vi "control loop bookkeeping.vi"(4 "worker pool reference":T2, 6 "fault fifo":refnum<k33>, 8 "engine error in":errorcluster, 9 "status reporting in":T19={"late? index (bool)"=-1, "late count index (U32)"=-1, "dt (ns) index (U64)"=-1}, 10 "time data in":T1, 11 "control loop data in":T5 {"module information"."GUID"."Lo" format="%.0x"; "module information"."GUID"."Hi" format="%.0x"}) -> (0 "engine error out":errorcluster, 1 "safe state?":bool, 2 "time data out":T1, 3 "control loop data out":T5 {"module information"."GUID"."Lo" format="%.0x"; "module information"."GUID"."Hi" format="%.0x"})   [LabVIEW 2013, in "main engine.lvlib"]
doc: "This VI writes to any of the timing or error tags that have been configured based on the results of this iteration of the loop."
uses:
  main engine/main engine.lvlib
  status reporting data.ctl
  control loop data.ctl
  <vilib>/NI/Tag Bus/table/data table.ctl
  engine run schedule.ctl
  engine decimation schedule.ctl
  full module data.ctl
  <vilib>/NI/Tag Bus Module Framework/runtime/TBM module execution interface.lvclass
  module run state.ctl
  async executor/asynchronous executor reference.ctl
  async executor/message to executor.ctl
  async command notification.ctl
  async error info.ctl
  <vilib>/NI/Tag Bus Module Framework/runtime/error classification.ctl
  <vilib>/NI/Tag Bus/buffer exchange/buffer reference.ctl
  <vilib>/NI/Tag Bus Module Framework/module configuration/TBM module configuration.lvclass
  <vilib>/NI/Configuration Framework/serializable configuration/Numeric GUID.ctl
  module method data.ctl
  <vilib>/NI/Tag Bus/table/transfer specification.ctl
  <vilib>/NI/Tag Bus/tag/Data Type.ctl
  fault handling spec.ctl
  Configuration/Error Actions.ctl
  rt fault.ctl
  worker library/worker comms.ctl
  worker library/worker commands.ctl
  worker library/request fifos.ctl
  worker library/recovery request.ctl
  worker library/response fifos.ctl
  worker library/recovery response.ctl
  time information.ctl
  <vilib>/NI/Tag Bus/table/write data element.vi
  <vilib>/NI/Tag Bus/table/data polymorphs/write one/write I32.vi
  perform asynchronous fault handling.vi
  perform fault handling.vi
  <vilib>/NI/Tag Bus/table/data polymorphs/write one/write Boolean.vi
  <vilib>/NI/Tag Bus/table/data polymorphs/write one/write U32.vi
  <vilib>/NI/Tag Bus/table/data polymorphs/write one/write U64.vi
  rt swap object in dvr.vi
  worker library/request recovery.vi
  <vilib>/NI/Tag Bus/table/data table.lvlib
  <vilib>/NI/Tag Bus/tag/tag descriptor.lvclass
  Configuration/Standard Engine Configuration.lvclass
  <vilib>/NI/Tag Bus/buffer exchange/tag bus buffer exchange.lvlib
  async executor/async executor.lvlib
  <vilib>/NI/Configuration Framework/serializable configuration/NISE_CEF_serializable configuration.lvclass
  worker library/worker pool.lvlib
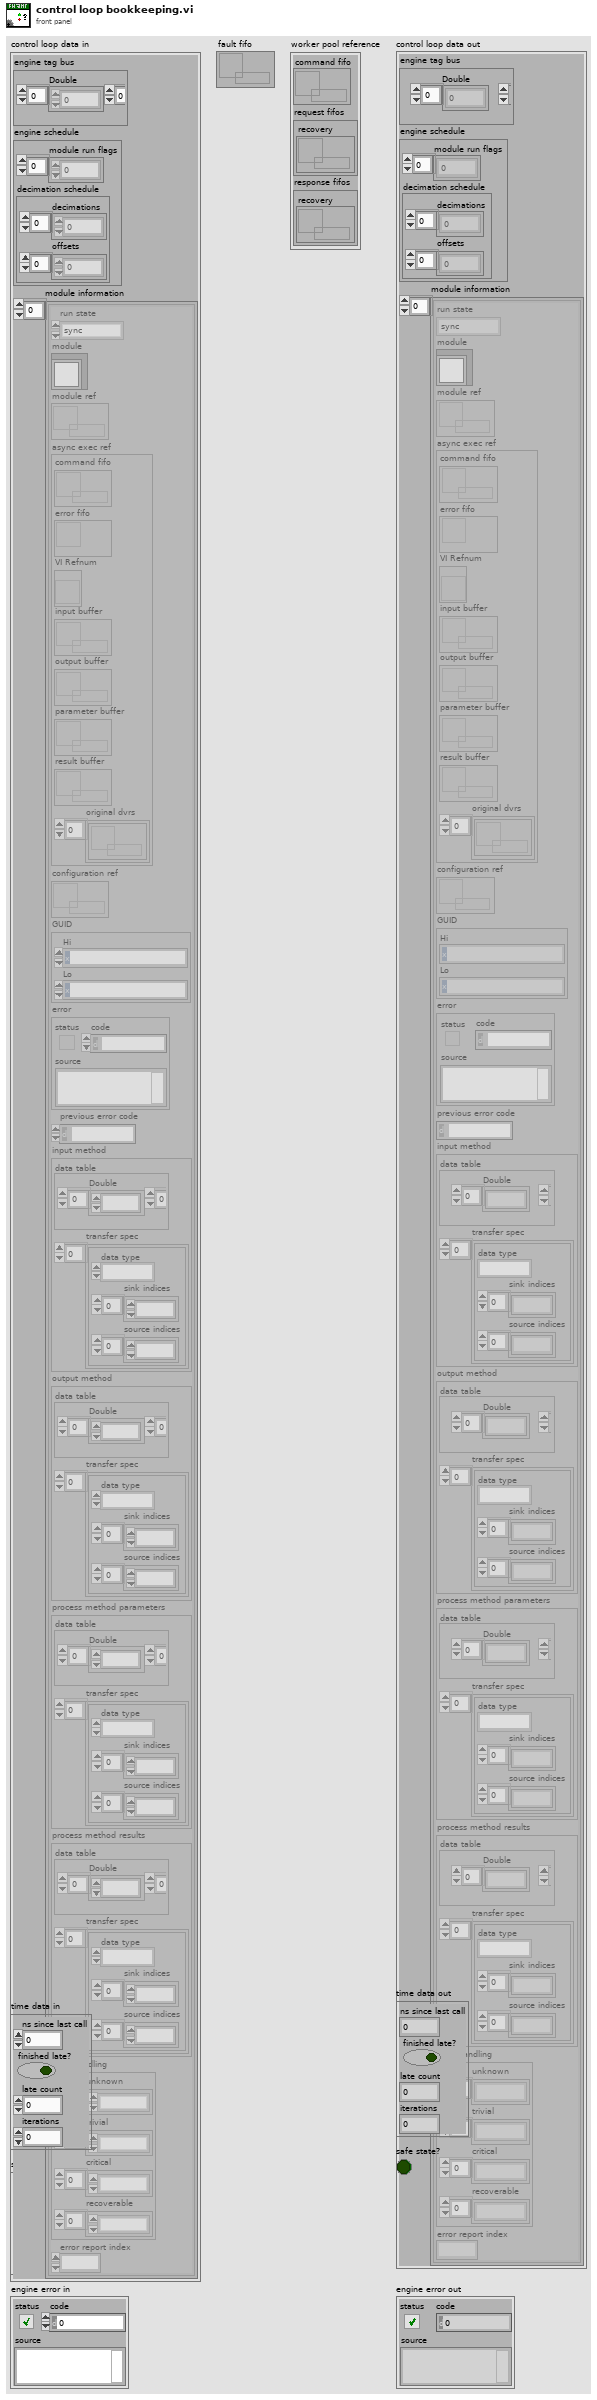
[diagram p1: front panel]
types:
  T1 = typedef "main engine.lvlib/time information.ctl" = cluster{"ns since last call":u64, "finished late?":bool, "late count":u32, "iterations":u64}
  T2 = typedef "worker pool.lvlib/worker comms.ctl" = cluster{"command fifo":refnum<k33>, "request fifos":T3, "response fifos":T4}
  T3 = typedef "worker pool.lvlib/request fifos.ctl" = cluster{"recovery":refnum<k33>}
  T4 = typedef "worker pool.lvlib/response fifos.ctl" = cluster{"recovery":refnum<k33>}
  T5 = typedef "main engine.lvlib/control loop data.ctl" = cluster{"engine tag bus":T6, "engine schedule":T7, "module information":T9[]}
  T6 = typedef "tag bus.lvlib/data table.lvlib/data table.ctl" = cluster{"Double":dbl[], "Single":sgl[], "I64":i64[], "I32":i32[], "I16":i16[], "I8":i8[], "U64":u64[], "U32":u32[], "U16":u16[], "U8":u8[], "Boolean":bool[], "String":string[], "Array of Double":cluster{"DBL Array":dbl[]}[], "Array of Single":cluster{"SGL Array":sgl[]}[], "Array of I64":cluster{"I64 Array":i64[]}[], "Array of I32":cluster{"I32 Array":i32[]}[], "Array of I16":cluster{"I16 Array":i16[]}[], "Array of I8":cluster{"I8 Array":i8[]}[], "Array of U64":cluster{"U64 Array":u64[]}[], "Array of U32":cluster{"U32 Array":u32[]}[], "Array of U16":cluster{"U16 Array":u16[]}[], "Array of U8":cluster{"U8 Array":u8[]}[], "Array of Boolean":cluster{"Boolean Array":bool[]}[], "Array of String":cluster{"String Array":string[]}[]}
  T7 = typedef "main engine.lvlib/engine run schedule.ctl" = cluster{"module run flags":u8[], "decimation schedule":T8}
  T8 = typedef "main engine.lvlib/engine decimation schedule.ctl" = cluster{"decimations":u16[], "offsets":u16[]}
  T9 = typedef "main engine.lvlib/full module data.ctl" = cluster{"run state":T10, "module":refnum<class "TBM module execution interface.lvclass">, "module ref":refnum<data-value>, "async exec ref":T11, "configuration ref":refnum<data-value>, "GUID":T13, "error":errorcluster, "previous error code":i32, "input method":T14, "output method":T14, "process method parameters":T14, "process method results":T14, "fault handling":T17, "error report index ":i32}
  T10 = typedef "main engine.lvlib/module run state.ctl" = enum16{"sync", "async"}
  T11 = typedef "async executor.lvlib/asynchronous executor reference.ctl" = cluster{"command fifo":refnum<k33>, "error fifo":refnum<k33>, "VI Refnum":refnum<vi>, "input buffer":refnum<k33>, "output buffer":refnum<k33>, "parameter buffer":refnum<k33>, "result buffer":refnum<k33>, "original dvrs":T12[]}
  T12 = typedef "tag bus buffer exchange.lvlib/buffer reference.ctl" = refnum<data-value>
  T13 = typedef "NISE_CEF_serializable configuration.lvclass/Numeric GUID.ctl" = cluster{"Hi":u64, "Lo":u64}
  T14 = typedef "main engine.lvlib/module method data.ctl" = cluster{"data table":T6, "transfer spec":T15[]}
  T15 = typedef "tag bus.lvlib/data table.lvlib/transfer specification.ctl" = cluster{"data type":T16, "sink indices":i32[], "source indices":i32[]}
  T16 = typedef "tag bus.lvlib/tag descriptor.lvclass/Data Type.ctl" = enum16{"Double", "Single", "I64", "I32", "I16", "I8", "U64", "U32", "U16", "U8", "Boolean", "String", "Array of Double", "Array of Single", "Array of I64", "Array of I32", "Array of I16", "Array of I8", "Array of U64", "Array of U32", "Array of U16", "Array of U8", "Array of Boolean", "Array of String"}
  T17 = typedef "main engine.lvlib/fault handling spec.ctl" = cluster{"unknown":T18[], "trivial":T18[], "critical":T18[], "recoverable":T18[]}
  T18 = typedef "Standard Engine Configuration.lvclass/Error Actions.ctl" = enum16{"Clear", "Notify", "Stop Component", "Stop Engine", "Safe State", "Attempt Recovery"}
  T19 = typedef "main engine.lvlib/status reporting data.ctl" = cluster{"late? index (bool)":i32, "late count index (U32)":i32, "dt (ns) index (U64)":i32}
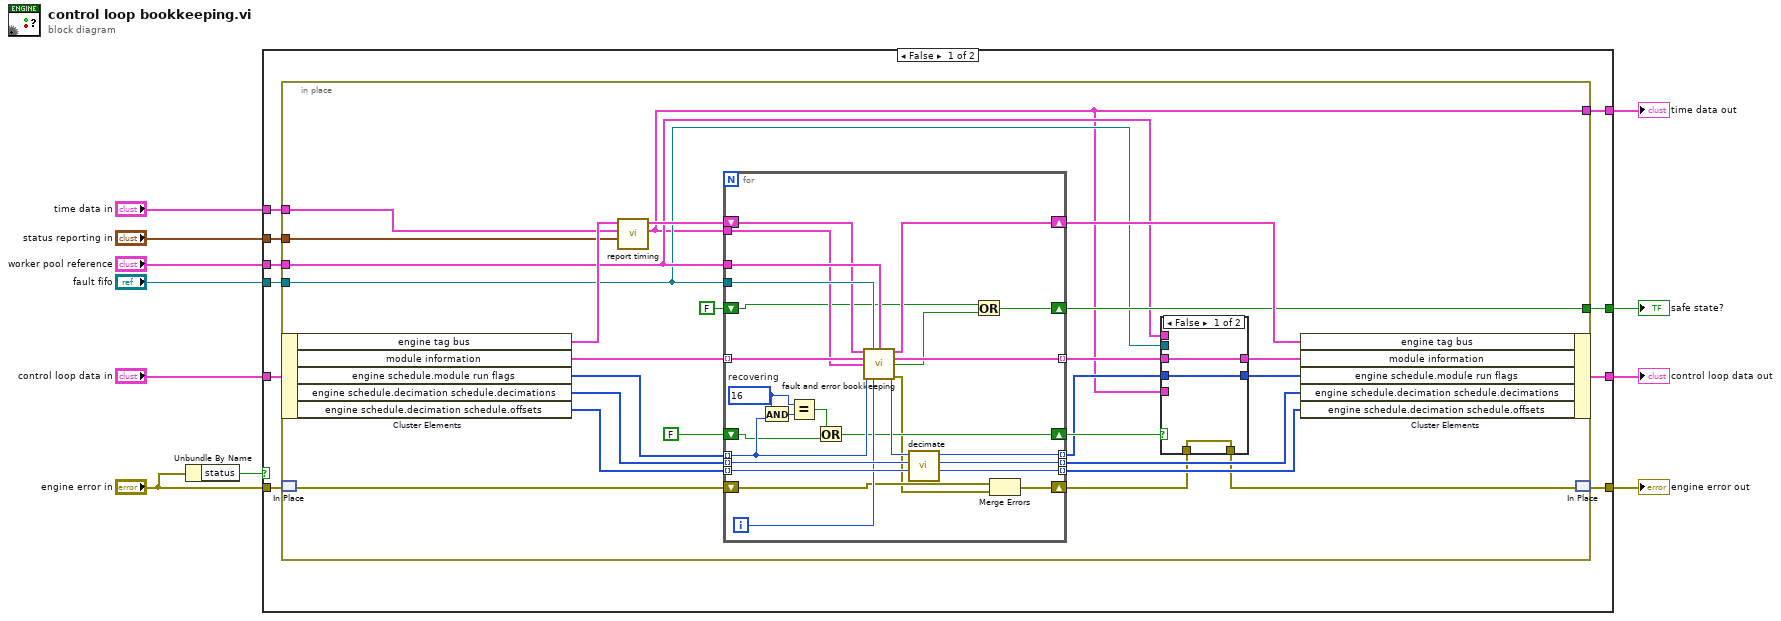
[diagram p0: block diagram]
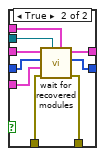
[diagram p2: hidden frame]
diagram:
  n1 = Unbundle By Name("engine error in") -> ("status"=w1:bool)
  n2 = case shown="False" w1 {
    tunnel: "control loop data in" -> [w21 w85]
    tunnel: [w20 w85] -> w10
    tunnel: "fault fifo" -> [w19 _]
    tunnel: "engine error in" -> [w18 w86]
    tunnel: [w17 w86] -> w8
    tunnel: "status reporting in" -> [w16 _]
    tunnel: "worker pool reference" -> [w15 _]
    tunnel: [w14 _] -> w5
    tunnel: [w13 w87] -> w4
    tunnel: "time data in" -> [w12 w87]
    frame False {
      n3 = in-place {
        in-place-border: [w23] -> w13
        in-place-border: w12 -> [w38]
        in-place-border: w19 -> [w26]
        in-place-border: w16 -> [w34]
        in-place-border: w15 -> [w27]
        in-place-border: [w35] -> w14
        n4 = in-place-cluster #1(w21) -> ("engine tag bus"=w39:T6, "module information"=w45:T9[], "engine schedule.module run flags"=w44:u8[], "engine schedule.decimation schedule.decimations"=w42:u16[], "engine schedule.decimation schedule.offsets"=w37:u16[])
        n5 = in-place-match #2(w18) -> (w41:errorcluster)
        n6 = call "report timing.vi"("status reporting tags"=w34, "time data in"=w38, "engine tag bus"=w39) -> ("time data out"=w23:T1, "engine data out"=w40:T6)  [unwired: 7 in]
        n7 = for {
          shift-right: [w75] -> w46
          shift-left: w40 -> [w76]
          tunnel: w45 -> [w73] mode=indexing
          tunnel: w44 -> [w67] mode=indexing
          tunnel: [w83] -> w29 mode=indexing
          tunnel: [w82] -> w43 mode=indexing
          tunnel: [w81] -> w36 mode=indexing
          tunnel: w42 -> [w79] mode=indexing
          tunnel: w37 -> [w78] mode=indexing
          tunnel: w26 -> [w84]
          shift-right: [w59] -> w25
          shift-left: w41 -> [w61]
          tunnel: w27 -> [w77]
          tunnel: [w74] -> w31 mode=indexing
          tunnel: w23 -> [w71]
          shift-right: [w65] -> w32
          shift-left: FALSE -> [w64]
          shift-right: [w63] -> w35
          shift-left: FALSE ("safe state?") -> [w62]
          i -> [w70]
          w69 = u8 16  # recovering
          n8 = And(x=w69, y=w67) -> (x .and. y?=w68:u8)
          n9 = Equal?(x=w69, y=w68) -> (x = y?=w66:bool)
          n10 = Or(x=w66, y=w64) -> (x .or. y?=w65:bool)
          n11 = call "fault and error bookkeeping.vi"("data table in"=w76, "fault fifo"=w84, "worker pool reference"=w77, "module data"=w73, "time data in"=w71, "run flags in"=w67, "module index"=w70) -> ("data table out"=w75:T6, "module data out"=w74:T9, "safe state?"=w72:bool, "run flags out"=w80:u8, "engine error out"=w60:errorcluster)  [unwired: 4 in]
          n12 = call "decimate.vi"("offset"=w78, "decimation"=w79, "run flags"=w80) -> ("new offset"=w81:u16, "decimation out"=w82:u16, "run flags out"=w83:u8)  [unwired: 6 in]
          n13 = Or(x=w62, y=w72) -> (x .or. y?=w63:bool)
          n14 = Merge Errors(w61, w60) -> (w59:errorcluster)
        }
        n15 = case shown="False" w32 {
          tunnel: w31 -> [w49 w57]
          tunnel: [w49 w58] -> w30
          tunnel: w29 -> [w48 w56]
          tunnel: [w48 w55] -> w28
          tunnel: w27 -> [_ w54]
          tunnel: w26 -> [_ w53]
          tunnel: w25 -> [w47 w52]
          tunnel: [w47 w51] -> w24
          tunnel: w23 -> [_ w50]
          frame False {
          }
          frame True {
            n16 = call "wait for recovered modules.vi"("worker pool reference"=w54, "fault fifo"=w53, "error in"=w52, "time data in"=w50, "run flags in"=w56, "modules in"=w57) -> ("error out"=w51:errorcluster, "run flags out"=w55:u8[], "modules out"=w58:T9[])  [unwired: 3 in]
          }
        }
        n17 = in-place-cluster #1("engine tag bus"=w46, "module information"=w30, "engine schedule.module run flags"=w28, "engine schedule.decimation schedule.decimations"=w43, "engine schedule.decimation schedule.offsets"=w36) -> (w20:T5)
        n18 = in-place-match #2(w24) -> (w17:errorcluster)
      }
    }
    frame True {
    }
  }
  "control loop data out" <- w10
  "engine error out" <- w8
  "safe state?" <- w5
  "time data out" <- w4
